vi "Initialize DAQmx References.vi"(8 "error in (no error)":errorcluster, 10 "Hardware Config Cluster":T1 {"Unit" items=["Volts", "From Custom Scale"]}, 11 "Task Name":string) -> (0 "error out":errorcluster, 2 "Hardware Config Cluster Out":T1 {"Unit" items=["Volts", "From Custom Scale"]}, 3 "HW Refnum Out":string)   [LabVIEW 2020, in "Acquisition.lvlib"]
uses:
  Acquisition.lvlib
  Settings Editor/DAQmx Config--cluster.ctl
  <vilib>/DAQmx/create/channels.llb/DAQmx Create Channel (AI-Voltage-Basic).vi
  Settings Editor/Settings Editor.lvlib
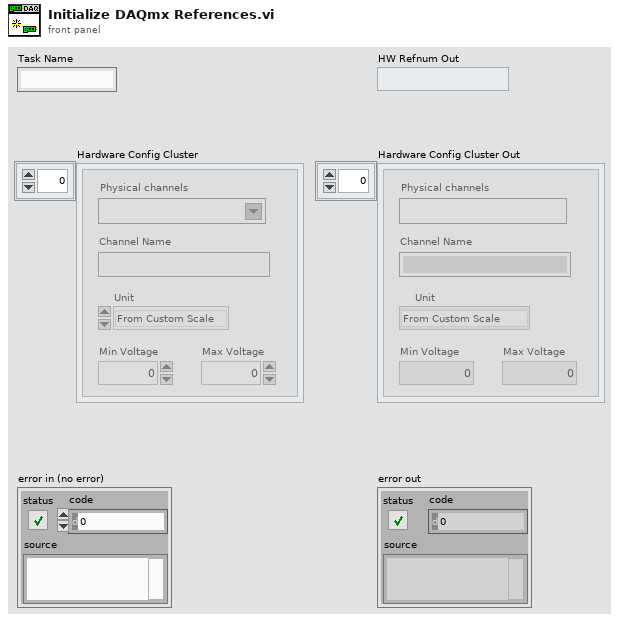
[diagram p1: front panel]
types:
  T1 = typedef "Settings Editor.lvlib/DAQmx Config--cluster.ctl" = cluster{"Physical channels":tag, "Channel Name":string, "Unit":i32, "Min Voltage":dbl, "Max Voltage":dbl}[]
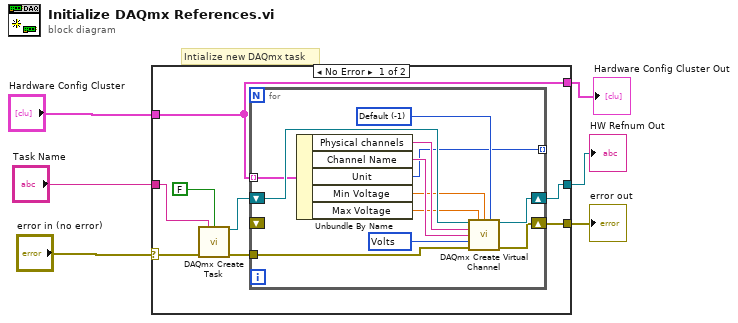
[diagram p0: block diagram]
diagram:
  # "Intialize new DAQmx task"
  n1 = case shown="No Error" "error in (no error)" {
    selector: "error in (no error)" -> [w8 w28]
    tunnel: "Task Name" -> [w12 w29]
    tunnel: "Hardware Config Cluster" -> [w7 w27]
    tunnel: [w10 w28] -> w4
    tunnel: [w9 w29] -> w3
    tunnel: [w7 w27] -> w1
    frame No Error {
      n2 = call <vilib>:"DAQmx Create Task.vi"("new task name"=w12, "auto cleanup"=FALSE, "error in"=w8) -> ("task out"=w14:refnum<k21>, "error out"=w11:errorcluster)  [unwired: 11 in]
      n3 = for {
        shift-right: [w25] -> w9
        shift-left: w14 -> [w26]
        tunnel: w11 -> [w24]
        shift-right: [w23] -> w10
        shift-left: _ -> [_]
        tunnel: [w18] -> _ mode=indexing
        tunnel: w7 -> [w15] mode=indexing
        w21 = 10348 items=["Volts"=10348, "From Custom Scale"=10065] ("units")
        w22 = -1 items=["Default"=-1, "RSE"=10083, "NRSE"=10078, "Differential"=10106, "Pseudodifferential"=12529] ("input terminal configuration")
        n4 = Unbundle By Name(w15) -> ("Physical channels"=w20:tag, "Channel Name"=w19:string, "Unit"=w18:i32, "Min Voltage"=w17:dbl, "Max Voltage"=w16:dbl)
        n5 = call-poly <vilib>:"DAQmx Create Virtual Channel.vi"("task in"=w26, "maximum value"=w16, "minimum value"=w17, "input terminal configuration"=w22, "physical channels"=w20, "name to assign"=w19, "units"=w21, "error in"=w24) -> ("task out"=w25:refnum<k21>, "error out"=w23:errorcluster)  [unwired: 6 in]
      }
    }
    frame Error {
    }
  }
  "error out" <- w4
  "HW Refnum Out" <- w3
  "Hardware Config Cluster Out" <- w1
